vi "Check if Folder exists.vi"(8 "error in (no error)":errorcluster, 11 "Exp Params in":T1 {"period" min=1; "total stacks" min=1; "images per stack" min=1; "total images" min=1; "Z Stack Settings"."Start" min=0.0 max=100.0 step=0.1; "Z Stack Settings"."Step Size" min=0.1 max=100.0 step=0.1; "Z Stack Settings"."Finish" min=0.0 max=100.0 step=0.1; "TSFrames" min=1 step=1; "ZTSdt" min=1 step=1; "ZTSFrames" min=2 step=1; "TSfps" min=1 max=1000 step=1}) -> (0 "error out":errorcluster, 3 "Exp Params out":T1 {"period" min=1; "total stacks" min=1; "images per stack" min=1; "total images" min=1; "Z Stack Settings"."Start" min=0.0 max=100.0 step=0.1; "Z Stack Settings"."Step Size" min=0.1 max=100.0 step=0.1; "Z Stack Settings"."Finish" min=0.0 max=100.0 step=0.1; "TSFrames" min=1 step=1; "ZTSdt" min=1 step=1; "ZTSFrames" min=2 step=1; "TSfps" min=1 max=1000 step=1})   [LabVIEW 2020]
uses:
  _Controls/Exp Params.ctl
  _Globals/Global Controls.vi
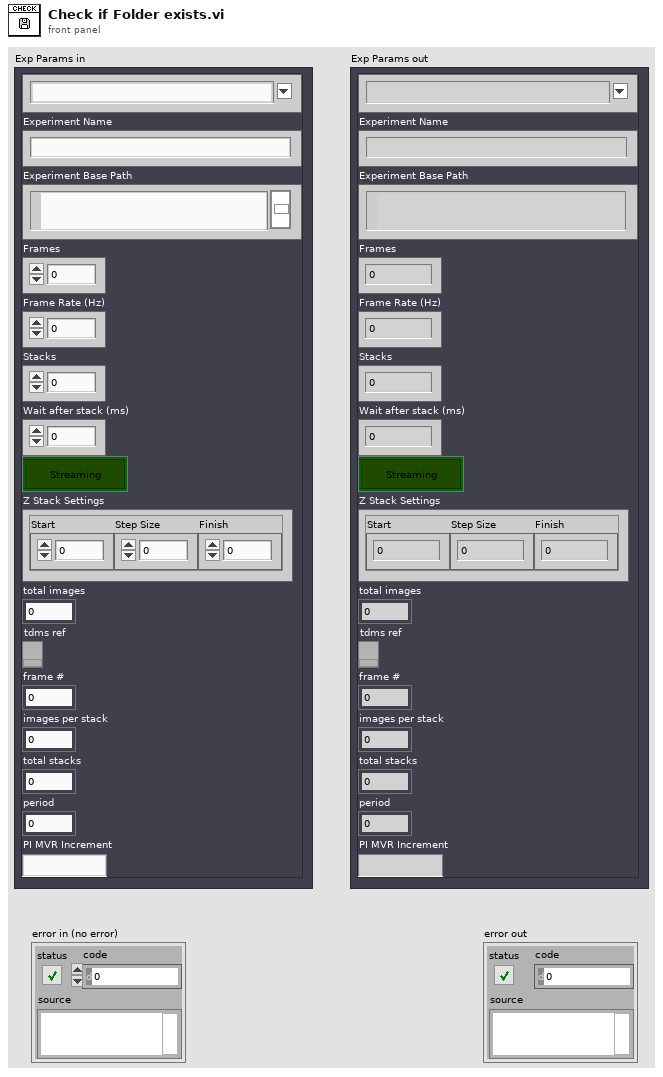
[diagram p1: front panel]
types:
  T1 = typedef "Exp Params.ctl" = cluster{"Experiment Type":string, "Experiment Name":string, "ExpPath":path, "TSFrames":i32, "TSfps":i32, "ZTSFrames":i32, "ZTSdt":i32, "Streaming":bool, "Z Stack Settings":cluster{"Start":dbl, "Step Size":dbl, "Finish":dbl}, "total images":i32, "tdms ref":refnum<k34>, "frame #":i64, "images per stack":i32, "total stacks":i32, "period":i32, "PI MVR Increment":string}
  T2 = enum16{"open", "open or create", "create or replace", "create", "open (read-only)"}
  T3 = typedef "Tweezertron Ctrl Refs.ctl" = cluster{"LSM Settings":refnum<vi>, "iFlex Control":refnum<vi>, "PIFOC Settings":refnum<vi>, "PinSelector":refnum<vi>, "Manlight Controls":refnum<vi>, "Exp Params":refnum<vi>, "Image Thresholds":refnum<vi>, "RevFrame":refnum<vi>, "Spots":refnum<vi>}
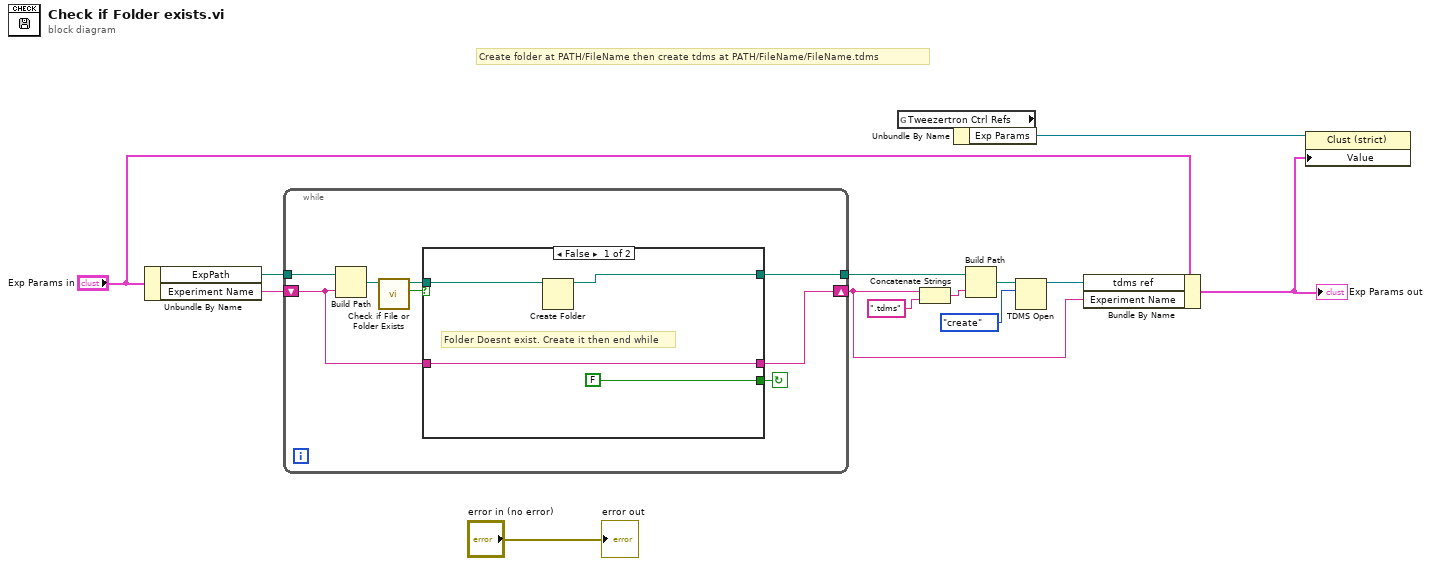
[diagram p0: block diagram]
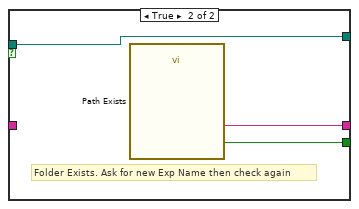
[diagram p2: hidden frame]
diagram:
  # "Create folder at PATH/FileName then create tdms at PATH/FileName/FileName.tdms"
  n1 = Unbundle By Name("Exp Params in") -> ("ExpPath"=w4:path, "Experiment Name"=w6:string)
  n2 = while {
    tunnel: [w18] -> w5
    shift-right: [w16] -> w1
    shift-left: w6 -> [w15]
    tunnel: w4 -> [w17]
    stop <- w20 continue-if-true
    n3 = Build Path(base path=w17, name or relative path=w15) -> (appended path=w19:path)
    n4 = call <vilib>:"Check if File or Folder Exists.vi"("path"=w19) -> ("file or folder exists?"=w22:bool, "dup path"=w21:path)  [unwired: 8 in, 1 out]
    n5 = case shown="False" w22 {
      tunnel: w21 -> [w26 w27]
      tunnel: [FALSE ("Rename") w29] -> w20
      tunnel: [w25 w27] -> w18
      tunnel: [w24 w28] -> w16
      tunnel: w15 -> [w24 _]
      frame False {
        # "Folder Doesnt exist. Create it then end while"
        n6 = Create Folder(path (use dialog)=w26) -> (created path=w25:path)  [unwired: 2 in, 2 out]
      }
      frame True {
        # "Folder Exists. Ask for new Exp Name then check again"
        n7 = call "Path Exists"() -> ("NewName"=w28:string, "Rename"=w29:bool)  [unwired: 17 in, 1 out]
      }
    }
  }
  n8 = global read "Global Controls.vi" "Tweezertron Ctrl Refs"() -> (w9:T3)
  n9 = Concatenate Strings(w1, ".tdms" ("string")) -> (w12:string)
  n10 = Unbundle By Name(w9) -> ("Exp Params"=w8:refnum<vi>)
  n11 = Build Path(base path=w5, name or relative path=w12) -> (appended path=w11:path)
  n12 = TDMS Open(10:T2."create" ("operation (0:open)"), 11:w11) -> (3:w13:refnum<k34>)  [unwired: 5 in, 1 out]
  n13 = Bundle By Name(cluster="Exp Params in", "tdms ref"=w13, "Experiment Name"=w1) -> (w3:T1)
  "Exp Params out" <- w3
  n14 = property class="Clust (strict)"(reference=w8, "Value"=w3) -> ()  [unwired: 1 in, 2 out]
  "error out" <- "error in (no error)"
